vi "保存模版.vi"() -> ()   [LabVIEW 2018]
panel:
  out "保存模版":sgl[][](array[numeric])
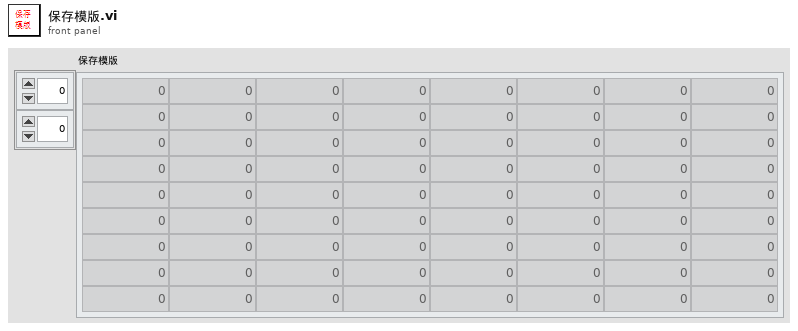
[diagram p1: front panel]
types:
  T1 = cluster{"Fx":sgl[], "Fy":sgl[], "Dx":sgl[], "Dy":sgl[]}
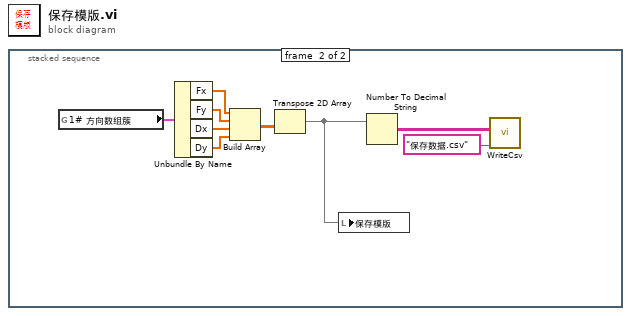
[diagram p0: block diagram]
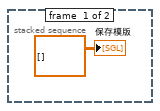
[diagram p2: hidden frame]
diagram:
  n1 = stacked-sequence {
    frame #0 {
      "保存模版" <- sgl[][] [] ("保存模版")
    }
    frame #1 {
      n2 = global read "全局 1.vi" "1# 方向数组簇"() -> (w10:T1)
      n3 = Unbundle By Name(w10) -> ("Fx"=w9:sgl[], "Fy"=w8:sgl[], "Dx"=w7:sgl[], "Dy"=w6:sgl[])
      n4 = Build Array(w9, w8, w7, w6) -> (w3:sgl[][])
      n5 = Transpose 2D Array(2D array=w3) -> (transposed array=w2:sgl[][])
      n6 = local write "保存模版"(w2) -> ()
      n7 = Number To Decimal String(number=w2) -> (decimal integer string=w5:string[][])  [unwired: 1 in]
      n8 = call "WriteCsv.vi"("相对路径"="保存数据.csv", "2D data"=w5) -> ()  [unwired: 2 in, 1 out]
    }
  }
